vi "Render.vi"(7 "Renderer":refnum<class "Renderer.lvclass">, 8 "error in (no error)":errorcluster, 10 "Camera":refnum<class "Camera.lvclass">, 11 "Galaxy in":refnum<class "Galaxy.lvclass">) -> (0 "error out":errorcluster)   [LabVIEW 2021, in "Galaxy.lvclass"]
uses:
  Galaxy.lvclass
  Camera/Camera.lvclass
  Renderer/Renderer.lvclass
  Galaxy.lvclass/Galaxy.ctl
  LabSDL2/Source/Libraries/LibSDL2 Wrapper/LibSDL2.lvlib
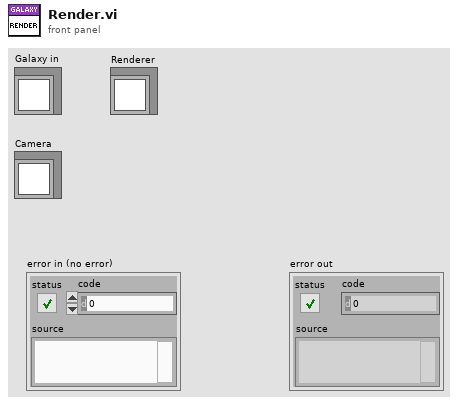
[diagram p1: front panel]
types:
  T1 = typedef "LibSDL2.lvlib/Rectangle.ctl" = cluster{"x":i32, "y":i32, "Width":i32, "Height":i32}
  T2 = typedef "Galaxy.lvclass/Star.ctl" = cluster{"Position":refnum<class "Vector 2D.lvclass">, "Texture Index":i32}
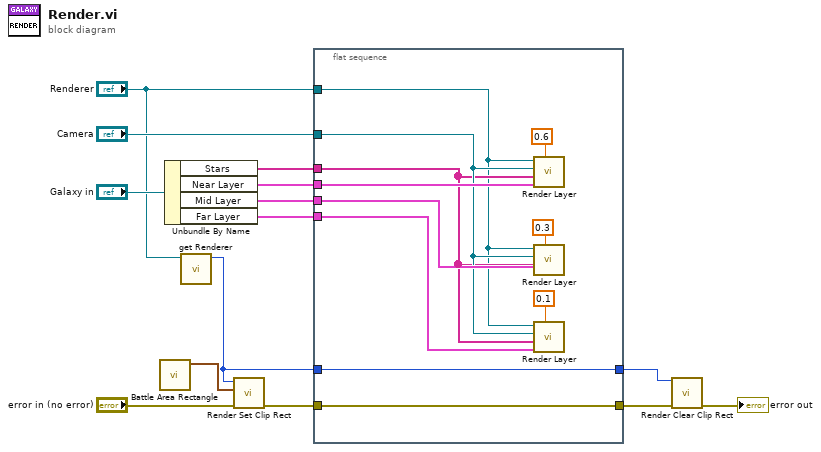
[diagram p0: block diagram]
diagram:
  n1 = call "Battle Area Rectangle.vi"() -> ("Viewport"=w1:T1)  [unwired: 11 in]
  n2 = Unbundle By Name("Galaxy in") -> ("Stars"=w9:string[], "Near Layer"=w11:T2[], "Mid Layer"=w12:T2[], "Far Layer"=w13:T2[])
  n3 = call-dynamic "get Renderer.vi"("Renderer in"="Renderer") -> ("Renderer"=w3:u32)  [unwired: 10 in]
  n4 = call "Render Set Clip Rect.vi"("error in"="error in (no error)", "Rectangle"=w1, "Renderer Pointer"=w3) -> ("error out"=w6:errorcluster)  [unwired: 7 in, 1 out]
  n5 = flat-sequence {
    tunnel: w13 -> [w25]
    tunnel: w12 -> [w24]
    tunnel: w11 -> [w23]
    tunnel: "Camera" -> [w22]
    tunnel: w9 -> [w21]
    tunnel: "Renderer" -> [w17]
    tunnel: w6 -> [w16]
    tunnel: [w16] -> w5
    tunnel: w3 -> [w15]
    tunnel: [w15] -> w2
    frame #0 {
      n6 = call "Render Layer.vi"("Factor"=0.6, "Layer"=w23, "Textures"=w21, "Camera"=w22, "Renderer in"=w17) -> ()  [unwired: 7 in]
      n7 = call "Render Layer.vi"("Factor"=0.3, "Layer"=w24, "Textures"=w21, "Camera"=w22, "Renderer in"=w17) -> ()  [unwired: 7 in]
      n8 = call "Render Layer.vi"("Factor"=0.1, "Layer"=w25, "Textures"=w21, "Camera"=w22, "Renderer in"=w17) -> ()  [unwired: 7 in]
    }
  }
  n9 = call "Render Clear Clip Rect.vi"("error in"=w5, "Renderer Pointer"=w2) -> ("error out"=→"error out":errorcluster)  [unwired: 8 in, 1 out]
